vi "Configure.vi"(8 "error in":errorcluster, 10 "name":string="nCRDS", 11 "nCRD in":refnum<class "gCRD.lvclass">) -> (0 "error out":errorcluster, 3 "nCRD out":refnum<class "gCRD.lvclass">)   [LabVIEW 2017, in "gCRDS.lvlib" / "gCRD.lvclass"]
doc: "Configures the CRDS for operation and starts all DAQmx tasks associated with the instrument. This VI overrides the parent VI in the Instrument class."
uses:
  gCRD.lvclass
  <vilib>/MSR Consulting, LLC/General Reuse/Instrument/Instrument.lvclass
  <vilib>/MSR Consulting, LLC/General Reuse/Instrument/state.ctl
  Session/Raw FPGA/FPGA Session.lvclass
  <vilib>/MSR Consulting, LLC/General Reuse/Session APIs/_Session Fwk/Session - Root.lvclass
  <vilib>/MSR Consulting, LLC/General Reuse/Session APIs/Session Log/System Log.lvclass
  <vilib>/MSR Consulting, LLC/General Reuse/CRDS/Main/CRDS.lvclass
  <vilib>/Utility/config.llb/NI_LVConfig.lvlib
  <vilib>/Utility/config.llb/Read Key (I32).vi
  Commands/Change Samples per Cycle/Change Samples per Cycle CMD.lvclass
  Commands/Change Rep Rate/Change Laser Rep Rate CMD.lvclass
  <vilib>/rvi/interface/nirviReadWriteControl/nirviReadWriteControl.xnode
  FPGA Ref.ctl
  <vilib>/MSR Consulting, LLC/General Reuse/Session APIs/File Access/Config Data/Config Data.lvclass
  <vilib>/MSR Consulting, LLC/General Reuse/CRDS/Cell/CRDS Cell.lvclass
  C:/Program Files (x86)/National Instruments/LabVIEW 2017/vi.lib/MSR Consulting, LLC/General Reuse/Instrument/Instrument.lvclass
  <vilib>/MSR Consulting, LLC/General Reuse/General/Math/Fit Exponential Class/Fit Exponential.lvclass
  C:/Program Files (x86)/National Instruments/LabVIEW 2017/vi.lib/MSR Consulting, LLC/General Reuse/Session APIs/_Session Fwk/Session - Root.lvclass
  C:/Program Files (x86)/National Instruments/LabVIEW 2017/vi.lib/MSR Consulting, LLC/General Reuse/Command/Command.lvclass
  FPGA Bitfiles/server_v1_2_2_5.lvbitx
  NiFpgaLv.dll
  <vilib>/Utility/error.llb/Error Cluster From Error Code.vi
  <vilib>/rvi/errors/niLvFpgaAdjustHostInterfaceError.vi
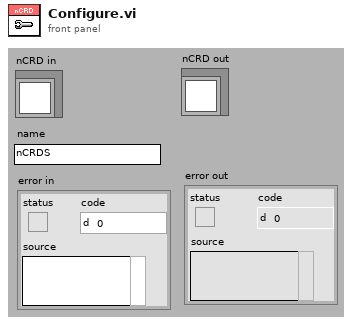
[diagram p1: front panel]
types:
  T1 = typedef "Instrument.lvclass/state.ctl" = enum8{"Configure", "Acquire", "Wait", "Quit", "Handle Error", "NOOP"}
  T2 = typedef "Session - Root.lvclass/Session Handle.ctl" = refnum<data-value>
  T3 = typedef "FPGA Ref.ctl" = refnum<k20>
  T4 = typedef "NI_LVConfig.lvlib/Config Data RefNum.ctl" = refnum<k1>
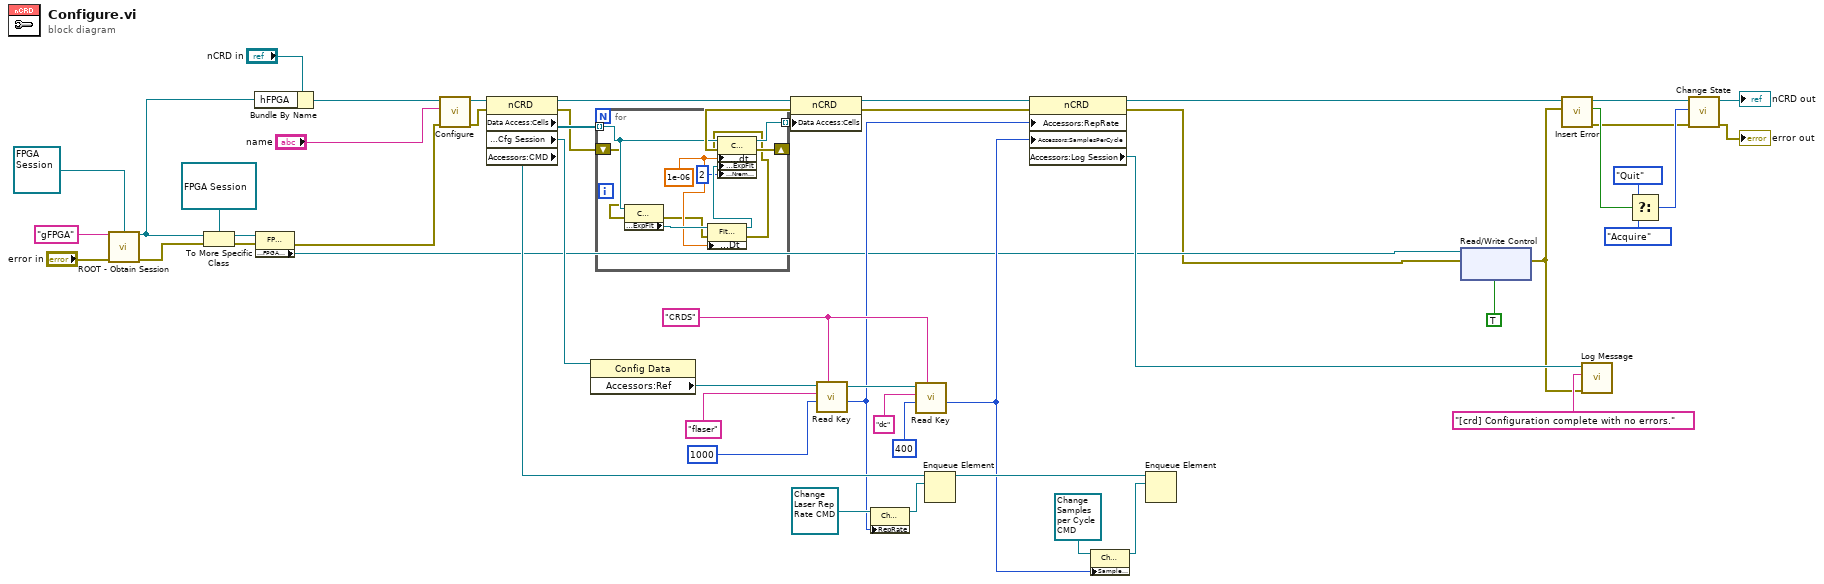
[diagram p0: block diagram]
diagram:
  w17 = "CRDS" ("section")
  n1 = call <vilib>:"ROOT - Obtain Session.vi"("Session Name ()"="gFPGA", "OBJ - Session"=refnum<class "FPGA Session.lvclass"> refnum ("FPGA Session.lvclass"), "error in (no error)"="error in") -> ("Session Handle"=w35:T2, "error out"=w34:errorcluster)  [unwired: 10 in, 1 out]
  n2 = To More Specific Class(target class=refnum<data-value> refnum ("hFPGA"), reference=w35, error in=w34) -> (specific class reference=w41:refnum<data-value>, error out=w33:errorcluster)
  n3 = Bundle By Name(cluster="nCRD in", "hFPGA"=w35) -> (w36:refnum<class "gCRD.lvclass">)
  n4 = property class="FPGA Session"(reference=w41, error in=w33) -> (error out=w40:errorcluster, "Accessors:FPGA Ref"=w2:T3)  [unwired: 1 out]
  n5 = call-parent "Configure.vi"("error in"=w40, "name"="name", "CRDS in"=w36) -> ("error out"=w28:errorcluster, "CRDS out"=w29:refnum<class "gCRD.lvclass">)  [unwired: 7 in]
  n6 = property class="nCRD"(reference=w29, error in=w28) -> (reference out=w25:refnum<class "gCRD.lvclass">, error out=w23:errorcluster, "Data Access:Cells"=w27:refnum<class "CRDS Cell.lvclass">[], "Accessors:Cfg Session"=w20:refnum<data-value>, "Accessors:CMD"=w12:refnum<queue>)
  n7 = property class="Config Data"(reference=w20) -> ("Accessors:Ref"=w19:T4)  [unwired: 1 in, 2 out]
  n8 = for {
    tunnel: w27 -> [w60] mode=indexing
    tunnel: [w62] -> w26 mode=indexing
    shift-right: [w61] -> w22
    shift-left: w23 -> [w56]
    w58 = 1e-06 ("dt")
    n9 = property class="CRDS Cell"(reference=w60, error in=w56) -> (error out=w55:errorcluster, "Accessors:ExpFit"=w59:refnum<class "Fit Exponential.lvclass">)  [unwired: 1 out]
    n10 = property class="Fit Exp"(reference=w59, error in=w55, "Accessors:Dt"=w58) -> (reference out=w57:refnum<class "Fit Exponential.lvclass">, error out=w54:errorcluster)
    n11 = property class="CRDS Cell"(reference=w60, error in=w54, "Accessors:dt"=w58, "Accessors:ExpFit"=w57, "Accessors:Nremove"=2 ("Nremove")) -> (reference out=w62:refnum<class "CRDS Cell.lvclass">, error out=w61:errorcluster)
  }
  n12 = property class="nCRD"(reference=w25, error in=w22, "Data Access:Cells"=w26) -> (reference out=w24:refnum<class "gCRD.lvclass">, error out=w21:errorcluster)
  n13 = call-poly <vilib>:"Read Key.vi"("section"=w17, "default value"=1000, "key"="flaser", "refnum"=w19) -> ("value"=w8:i32, "refnum out"=w16:T4)  [unwired: 4 in, 2 out]
  n14 = property class="Change Laser Rep Rate CMD"(reference=refnum<class "Change Laser Rep Rate CMD.lvclass"> refnum ("gCRDS.lvlib:Change Laser Rep Rate CMD"), "RepRate"=w8) -> (reference out=w9:refnum<class "Change Laser Rep Rate CMD.lvclass">)  [unwired: 1 in, 1 out]
  n15 = call-poly <vilib>:"Read Key.vi"("section"=w17, "default value"=400, "key"="dc", "refnum"=w16) -> ("value"=w7:i32)  [unwired: 4 in, 3 out]
  n16 = Enqueue Element(queue=w12, element=w9) -> (queue out=w11:refnum<queue>)  [unwired: 2 in, 2 out]
  n17 = property class="nCRD"(reference=w24, error in=w21, "Accessors:RepRate"=w8, "Accessors:SamplesPerCycle"=w7) -> (reference out=w49:refnum<class "gCRD.lvclass">, error out=w1:errorcluster, "Accessors:Log Session"=w31:T2)
  n18 = property class="Change Samples per Cycle CMD"(reference=refnum<class "Change Samples per Cycle CMD.lvclass"> refnum ("gCRDS.lvlib:Change Samples per Cycle CMD"), "SamplesperCycle"=w7) -> (reference out=w13:refnum<class "Change Samples per Cycle CMD.lvclass">)  [unwired: 1 in, 1 out]
  n19 = Enqueue Element(queue=w11, element=w13) -> ()  [unwired: 2 in, 3 out]
  n20 = xnode "Read/Write Control"("FPGA VI Reference In"=w2, "error in"=w1, "Transmit?"=TRUE) -> ("error out"=w5:errorcluster)  [unwired: 1 out]
  n21 = call <vilib>:"Insert Error.vi"("err"=w5, "Instrument in"=w49) -> ("error out"=w43:errorcluster, "error?"=w48:bool, "Instrument out"=w44:refnum<class "gCRD.lvclass">)  [unwired: 7 in]
  n22 = call <vilib>:"Log Message.vi"("error in"=w5, "MSG In"="[crd] Configuration complete with no errors.", "session in"=w31) -> ()  [unwired: 7 in, 2 out]
  n23 = Select(t=state."Quit" ("instr state"), s=w48, f=state."Acquire" ("instr state")) -> (s? t:f=w47:T1)
  n24 = call <vilib>:"Change State.vi"("error in"=w43, "instr state"=w47, "Instrument in"=w44) -> ("error out"=→"error out":errorcluster, "Instrument out"=→"nCRD out":refnum<class "gCRD.lvclass">)  [unwired: 7 in]
